vi "Clipboard 변환.vi"(2 "Input (structured)":string[][](table), 3 "Input (flattened)":string="1\t10\t100\n2\t11\t110\n3\t12\t120\n4\t13\t130\n5\t14\t140\n6\t15\t150\n7\t16\t160\n8\t17\t170\n9\t18\t180\n") -> (0 "Output (flattened)":string="1\t10\t100\n2\t11\t110\n3\t12\t120\n4\t13\t130\n5\t14\t140\n6\t15\t150\n7\t16\t160\n8\t17\t170\n9\t18\t180\n", 1 "Output (stuctured)":string[][](table))   [LabVIEW 2017]
panel:
  in  "탭 컨트롤":T1(tab)
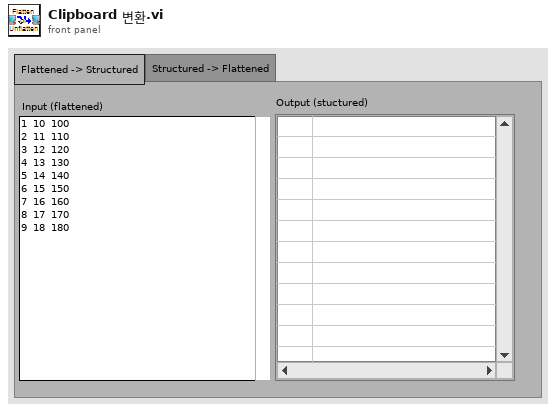
[diagram p1: front panel]
types:
  T1 = enum32{"Flattened -> Structured", "Structured -> Flattened"}
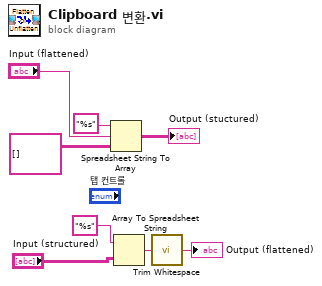
[diagram p0: block diagram]
diagram:
  n1 = Spreadsheet String To Array(format string="%s" ("포맷 문자열"), spreadsheet string="Input (flattened)", array type (2D Dbl)=string[][] [] ("배열 타입(2D Dbl)")) -> (array=→"Output (stuctured)":string[][])  [unwired: 1 in]
  n2 = Array To Spreadsheet String(array="Input (structured)", 3:"%s" ("포맷 문자열")) -> (spreadsheet string=w2:string)  [unwired: 1 in]
  n3 = call <vilib>:"Trim Whitespace.vi"("string"=w2) -> ("trimmed string"=→"Output (flattened)":string)  [unwired: 1 in]
